vi "evtDetailsToJSON.vi"(8 "error in (no error)":errorcluster, 9 "evtDetails":string="\"inPosition\" : True\n\"tolerance\" : 0.1\n\"position\" : [1,2,3]", 10 "evtName":string="move", 11 "TcpServer.lvclass":refnum<class "TcpServer.lvclass">) -> (0 "error out":errorcluster, 2 "JSON string":string, 3 "TcpServer.lvclass":refnum<class "TcpServer.lvclass">)   [LabVIEW 2018, in "TcpServer.lvclass"]
doc: "Convert the evtName and evtDetails in JSON string, to be sent to TCP Client.\n\nNOTE: Do not call this directly.This is for internal use only."
uses:
  TcpServer.lvclass
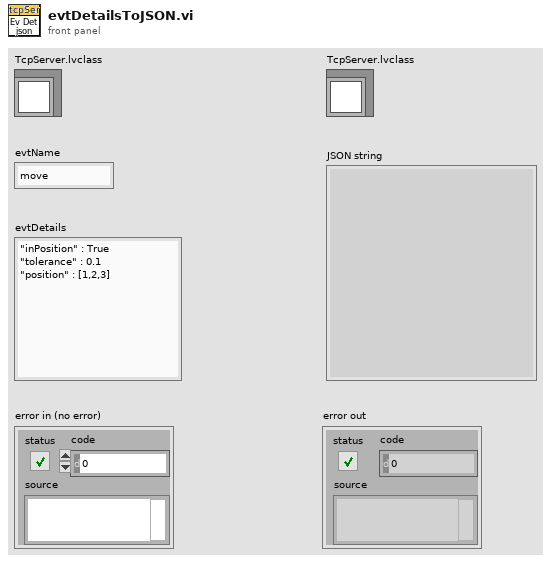
[diagram p1: front panel]
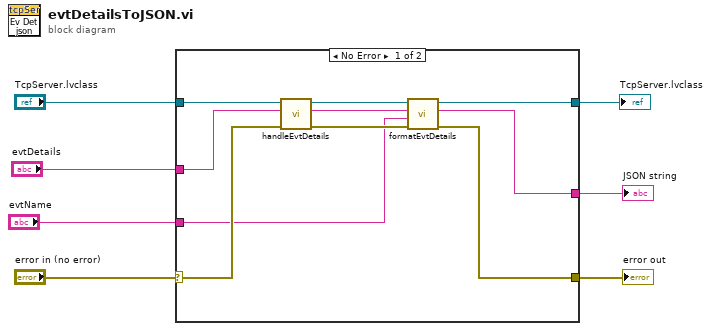
[diagram p0: block diagram]
diagram:
  n1 = case shown="No Error" "error in (no error)" {
    selector: "error in (no error)" -> [w11 w18]
    tunnel: "TcpServer.lvclass" -> [w16 w19]
    tunnel: [w14 w19] -> w6
    tunnel: "evtDetails" -> [w13 _]
    tunnel: "evtName" -> [w8 _]
    tunnel: [w12 _] -> w3
    tunnel: [w10 w18] -> w1
    frame No Error {
      n2 = call "handleEvtDetails.vi"("error in (no error)"=w11, "evtDetails"=w13, "TcpServer.lvclass"=w16) -> ("error out"=w17:errorcluster, "evtDetailsString"=w9:string, "TcpServer.lvclass"=w15:refnum<class "TcpServer.lvclass">)  [unwired: 6 in]
      n3 = call "formatEvtDetails.vi"("error in (no error)"=w17, "evtName"=w8, "evtDetailsString"=w9, "TcpServer.lvclass"=w15) -> ("error out"=w10:errorcluster, "jsonString"=w12:string, "TcpServer.lvclass"=w14:refnum<class "TcpServer.lvclass">)  [unwired: 5 in]
    }
    frame Error {
    }
  }
  "JSON string" <- w3
  "TcpServer.lvclass" <- w6
  "error out" <- w1
